vi "Normalize Angle.vi"(11 "Angle in r":dbl) -> (3 "Angle out r":dbl)   [LabVIEW 2020]
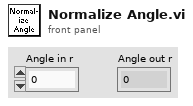
[diagram p1: front panel]
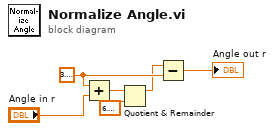
[diagram p0: block diagram]
diagram:
  w6 = 3.141592653589793
  n1 = Add(x=w6, y="Angle in r") -> (x+y=w2:dbl)
  n2 = Quotient & Remainder(x=w2, y=6.283185307179586) -> (x-y*floor(x/y)=w3:dbl)  [unwired: 1 out]
  n3 = Subtract(x=w3, y=w6) -> (x-y=→"Angle out r":dbl)
